vi "Add Rows (Variant).vi"(8 "error in (no error)":errorcluster, 9 "Data":variant[][](array[variant]), 11 "DataTable in":refnum<class "DataTable.lvclass">) -> (0 "error out":errorcluster, 3 "DataTable out":refnum<class "DataTable.lvclass">)   [LabVIEW 2016, in "DataGrid.lvlib" / "DataTable.lvclass"]
doc: "This allows any number of rows to be added to the datatable. The data must match the columns defined for the grid."
uses:
  <userlib>/LabVIEWdotNetDataGrid/source/DataTable/DataTable.lvclass
  <userlib>/LabVIEWdotNetDataGrid/source/DataTable/DataTable.lvclass/DataTable.ctl
  System.Data
  <userlib>/LabVIEWdotNetDataGrid/source/GridColumn/GridColumn.lvclass/GridColumn.ctl
  <userlib>/LabVIEWdotNetDataGrid/source/GridColumn/Read datatype.vi
  <userlib>/LabVIEWdotNetDataGrid/source/GridColumn/GridColumn.lvclass
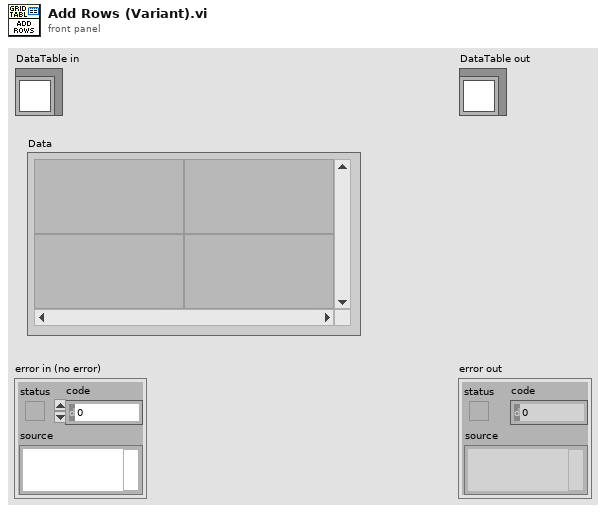
[diagram p1: front panel]
types:
  T1 = typedef "DataGrid.lvlib/GridColumn.lvclass/ColumnType.ctl" = enum16{"string", "image", "check", "numeric", "timestamp", "button", "combo", "link"}
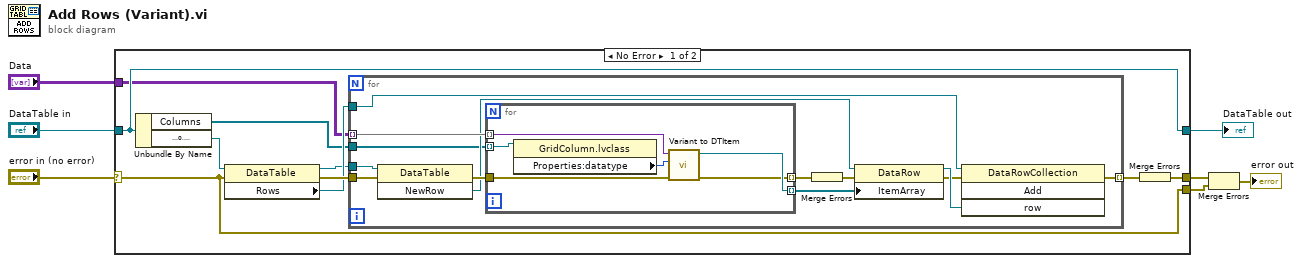
[diagram p0: block diagram]
diagram:
  n1 = case shown="No Error" "error in (no error)" {
    selector: "error in (no error)" -> [w13 w38]
    tunnel: [w13 w38] -> w6
    tunnel: [w14 w37] -> w4
    tunnel: "DataTable in" -> [w14 w37]
    tunnel: "Data" -> [w12 _]
    tunnel: [w10 _] -> w1
    frame No Error {
      n2 = Unbundle By Name(w14) -> ("Columns"=w9:refnum<class "GridColumn.lvclass">[], "DataTable"=w8:refnum<k24>)
      n3 = property class="DataTable"(reference=w8, error in=w13) -> (reference out=w11:refnum<k24>, error out=w17:errorcluster, "Rows"=w16:refnum<k24>)
      n4 = for {
        tunnel: w16 -> [w29]
        tunnel: w11 -> [w30]
        tunnel: [w28] -> w15 mode=indexing
        tunnel: w12 -> [w27] mode=indexing
        tunnel: w17 -> [w19]
        tunnel: w9 -> [w18]
        n5 = invoke class="DataTable" method="NewRow"(reference=w30, error in=w19) -> (error out=w26:errorcluster, "NewRow"=w25:refnum<k24>)  [unwired: 1 in, 1 out]
        n6 = for {
          tunnel: w27 -> [w32] mode=indexing
          tunnel: [w36] -> w23 mode=indexing
          tunnel: w26 -> [w35]
          tunnel: [w34] -> w22 mode=indexing
          tunnel: w18 -> [w33] mode=indexing
          n7 = property class="GridColumn.lvclass"(reference=w33) -> ("Properties:datatype"=w31:T1)  [unwired: 1 in, 2 out]
          n8 = call <userlib>:"Variant to DTItem.vi"("error in (no error)"=w35, "datatype"=w31, "element"=w32) -> ("error out"=w34:errorcluster, "DTItem .NET Refnum out"=w36:refnum<k24>)  [unwired: 7 in]
        }
        n9 = Merge Errors(w22) -> (w21:errorcluster)
        n10 = property class="DataRow"(reference=w25, error in=w21, "ItemArray"=w23) -> (reference out=w24:refnum<k24>, error out=w20:errorcluster)
        n11 = invoke class="DataRowCollection" method="Add"(reference=w29, error in=w20, "row"=w24) -> (error out=w28:errorcluster)  [unwired: 1 in, 3 out]
      }
      n12 = Merge Errors(w15) -> (w10:errorcluster)
    }
    frame Error {
    }
  }
  "DataTable out" <- w4
  n13 = Merge Errors(w1, w6) -> (→"error out":errorcluster)
